vi "TCP Connection.vi"(8 "error in (no error)":errorcluster, 11 "HTTP TCP Client in":refnum<class "HTTP TCP Client.lvclass">) -> (0 "error out":errorcluster, 2 "TCP Connection":refnum<k5>, 3 "HTTP TCP Client out":refnum<class "HTTP TCP Client.lvclass">)   [LabVIEW 2020, in "HTTP Server.lvlib" / "HTTP TCP Client.lvclass"]
uses:
  HTTP TCP Client.lvclass
  lv-stream-tcp/Stream-TCP/TCP Client/TCP Client.lvclass
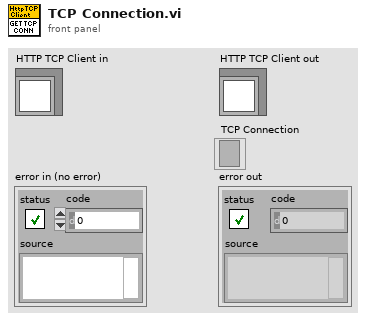
[diagram p1: front panel]
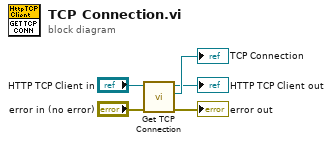
[diagram p0: block diagram]
diagram:
  n1 = call "Get TCP Connection.vi"("error in (no error)"="error in (no error)", "TCP Client in"="HTTP TCP Client in") -> ("error out"=→"error out":errorcluster, "TCP Connection"=→"TCP Connection":refnum<k5>, "TCP Client out"=→"HTTP TCP Client out":refnum<class "HTTP TCP Client.lvclass">)  [unwired: 7 in]
